vi "Save VIP Data.vi"(8 "Error In":errorcluster, 9 "Files Installed":path[](array[path]), 10 "Dependencies.config":path, 11 "Package Name":string) -> (0 "Error Out":errorcluster)   [LabVIEW 2011, in "LVH-Toolbox.lvlib" / "Installer Tools.lvlib"]
uses:
  Installer Tools.lvlib
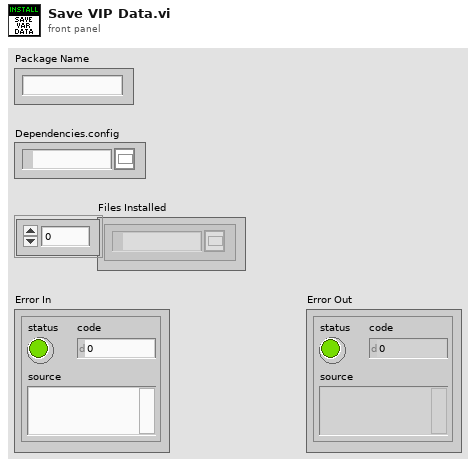
[diagram p1: front panel]
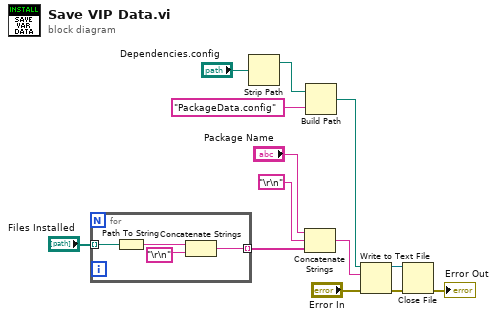
[diagram p0: block diagram]
diagram:
  n1 = for {
    tunnel: [w16] -> w5 mode=indexing
    tunnel: "Files Installed" -> [w15] mode=indexing
    n2 = Path To String(path=w15) -> (string=w17:string)
    n3 = Concatenate Strings(w17, "\r\n") -> (w16:string)
  }
  n4 = Strip Path(path="Dependencies.config") -> (stripped path=w12:path)  [unwired: 1 out]
  n5 = Concatenate Strings("Package Name", "\r\n", w5) -> (w3:string)
  n6 = Build Path(base path=w12, name or relative path="PackageData.config") -> (appended path=w1:path)
  n7 = Write to Text File(file (use dialog)=w1, text=w3, error in="Error In") -> (refnum out=w8:refnum<file>, error out=w9:errorcluster)  [unwired: 1 in, 1 out]
  n8 = Close File(refnum=w8, error in=w9) -> (error out=→"Error Out":errorcluster)  [unwired: 1 out]
